vi "mWADC_AVG_out.vi"(8 "error out":errorcluster, 11 "reference out":refnum<visa-resource-name>) -> (0 "error out 2":errorcluster, 2 "ADC_avg_out":i32, 3 "VISA resource name out":refnum<visa-resource-name>)   [LabVIEW 2019]
panel:
  out "Array":dbl[](array[numeric])
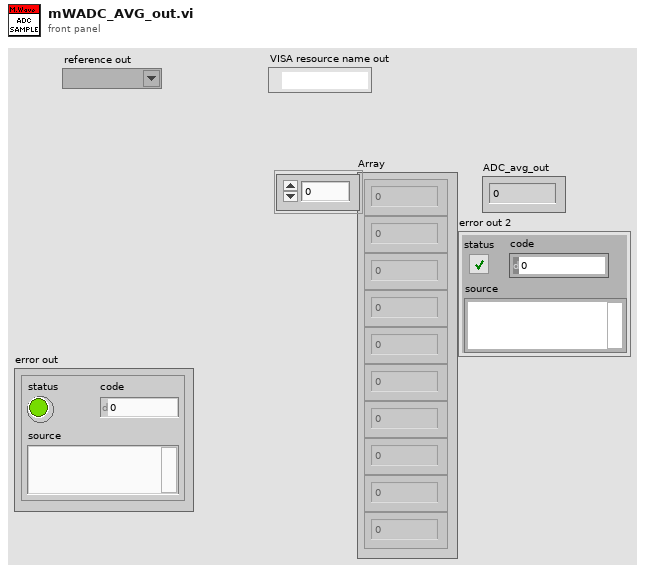
[diagram p1: front panel]
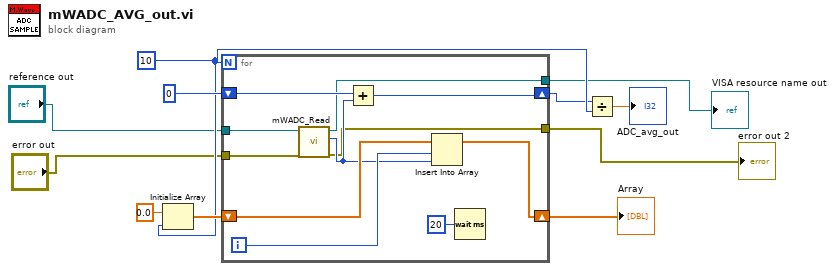
[diagram p0: block diagram]
diagram:
  w7 = 10
  n1 = Initialize Array(0.0 ("element"), w7) -> (w10:dbl[])
  n2 = for {
    N: w7 -> [_]
    tunnel: "reference out" -> [w22]
    tunnel: "error out" -> [w21]
    shift-right: [w18] -> w9
    shift-left: w10 -> [w19]
    shift-right: [w14] -> w6
    shift-left: 0 ("x") -> [w15]
    tunnel: [w13] -> w2
    tunnel: [w12] -> w1
    i -> [w20]
    n3 = call "mWADC_Read.vi"("error in (no error)"=w21, "MW_ADC"=w22) -> ("error out"=w13:errorcluster, "ADC Count"=w16:i32, "VISA resource name out"=w12:refnum<visa-resource-name>)  [unwired: 7 in]
    n4 = Add(x=w15, y=w16) -> (x+y=w14:i32)
    n5 = Insert Into Array(array=w19, index=w20, new element=w16) -> (w18:dbl[])
    n6 = Wait (ms)(milliseconds to wait=u32 20) -> ()  [unwired: 1 out]
  }
  "Array" <- w9
  "error out 2" <- w2
  "VISA resource name out" <- w1
  n7 = Divide(x=w6, y=w7) -> (x/y=→"ADC_avg_out":dbl)
